vi "WILT Start Stop Timer Set.vi"(4 "Station Number":i32, 6 "Injection Times":T1, 7 "Operation Type":T2=enum."Operate As Stand-Alone EXE", 10 "Inlet Timer":dbl, 11 "Station Test State In":T3) -> (3 "Outlet Timer":dbl)   [LabVIEW 2016]
uses:
  Type Definitions/WILT Station Test State Cluster.ctl
  Type Definitions/WILT Dryer Test State.ctl
  Type Definitions/WILT Water Valve EXE Operation Type.ctl
  Type Definitions/WILT Water Injection Control.ctl
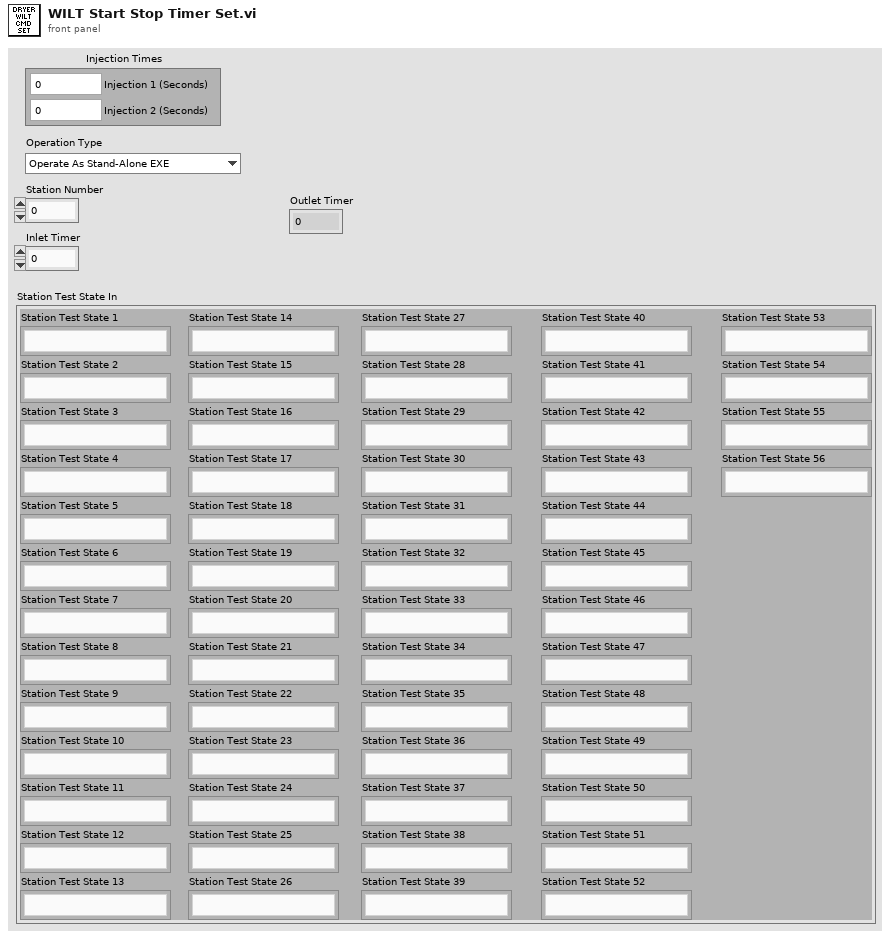
[diagram p1: front panel]
types:
  T1 = typedef "WILT Water Injection Control.ctl" = cluster{"Injection 1 (Seconds)":dbl, "Injection 2 (Seconds)":dbl}
  T2 = typedef "WILT Water Valve EXE Operation Type.ctl" = enum16{"Operate As SubVI", "Operate As Stand-Alone EXE", "Shutdown All Dryers"}
  T3 = typedef "WILT Station Test State Cluster.ctl" = cluster{"Station Test State 1":T4, "Station Test State 2":T4, "Station Test State 3":T4, "Station Test State 4":T4, "Station Test State 5":T4, "Station Test State 6":T4, "Station Test State 7":T4, "Station Test State 8":T4, "Station Test State 9":T4, "Station Test State 10":T4, "Station Test State 11":T4, "Station Test State 12":T4, "Station Test State 13":T4, "Station Test State 14":T4, "Station Test State 15":T4, "Station Test State 16":T4, "Station Test State 17":T4, "Station Test State 18":T4, "Station Test State 19":T4, "Station Test State 20":T4, "Station Test State 21":T4, "Station Test State 22":T4, "Station Test State 23":T4, "Station Test State 24":T4, "Station Test State 25":T4, "Station Test State 26":T4, "Station Test State 27":T4, "Station Test State 28":T4, "Station Test State 29":T4, "Station Test State 30":T4, "Station Test State 31":T4, "Station Test State 32":T4, "Station Test State 33":T4, "Station Test State 34":T4, "Station Test State 35":T4, "Station Test State 36":T4, "Station Test State 37":T4, "Station Test State 38":T4, "Station Test State 39":T4, "Station Test State 40":T4, "Station Test State 41":T4, "Station Test State 42":T4, "Station Test State 43":T4, "Station Test State 44":T4, "Station Test State 45":T4, "Station Test State 46":T4, "Station Test State 47":T4, "Station Test State 48":T4, "Station Test State 49":T4, "Station Test State 50":T4, "Station Test State 51":T4, "Station Test State 52":T4, "Station Test State 53":T4, "Station Test State 54":T4, "Station Test State 55":T4, "Station Test State 56":T4}
  T4 = typedef "WILT Dryer Test State.ctl" = enum16{"No Serial Number", "Waiting for Dryer To Start", "Drying Clothes", "Water Injection 1 (On)", "Water Injection 1 Timer", "Water Injection 1 (Off)", "Pause Dryer", "Sending Start Stop CMD", "Pause Dryer 2", "Sending Start Stop CMD 2", "Drying Clothes 2", "Water Injection 2 (On)", "Water Injection 2 Timer", "Water Injection 2 (Off)", "Drying Clothes 3", "Cooling Down", "Sending Start Stop CMD 3", "Increment Cycle"}
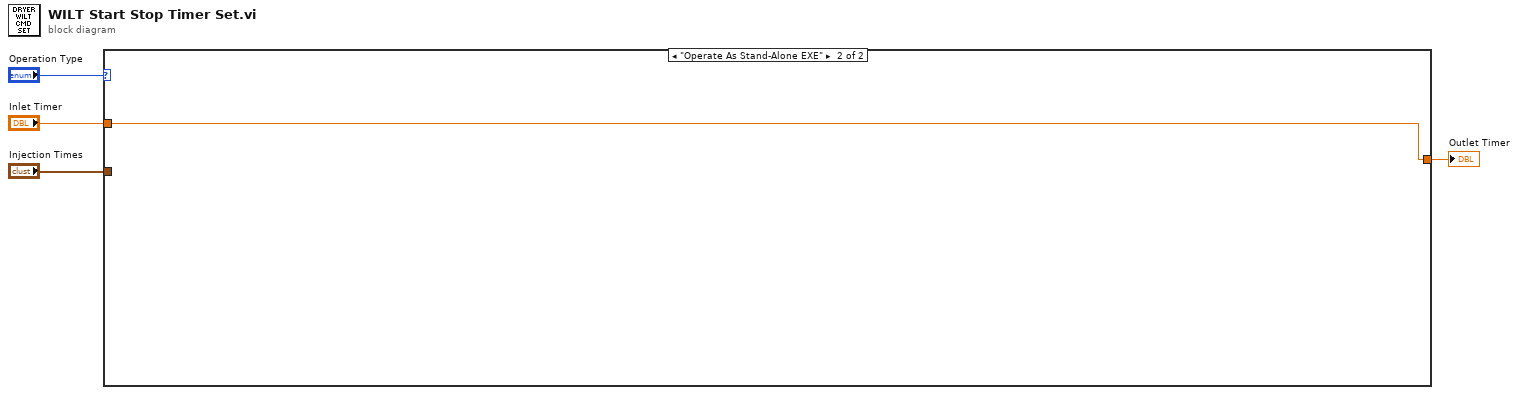
[diagram p0: block diagram]
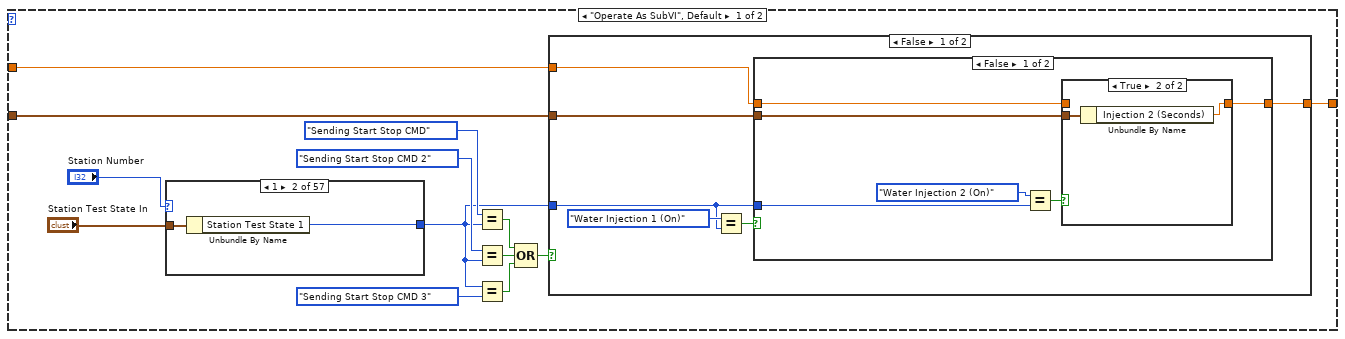
[diagram p2: hidden frame]
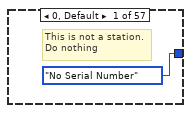
[diagram p3: hidden frame]
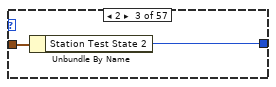
[diagram p4: hidden frame]
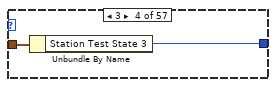
[diagram p5: hidden frame]
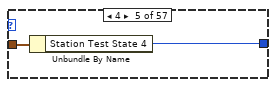
[diagram p6: hidden frame]
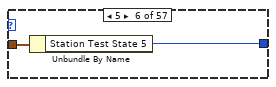
[diagram p7: hidden frame]
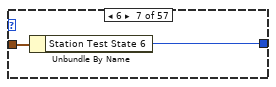
[diagram p8: hidden frame]
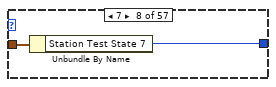
[diagram p9: hidden frame]
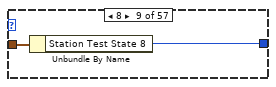
[diagram p10: hidden frame]
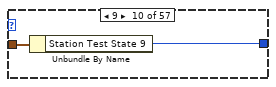
[diagram p11: hidden frame]
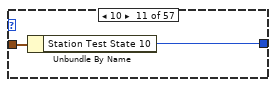
[diagram p12: hidden frame]
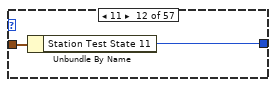
[diagram p13: hidden frame]
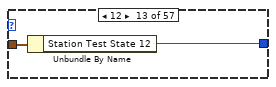
[diagram p14: hidden frame]
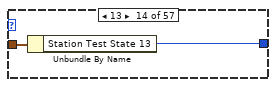
[diagram p15: hidden frame]
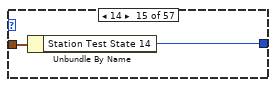
[diagram p16: hidden frame]
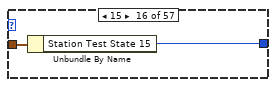
[diagram p17: hidden frame]
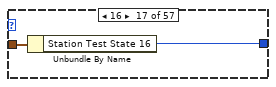
[diagram p18: hidden frame]
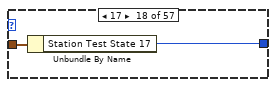
[diagram p19: hidden frame]
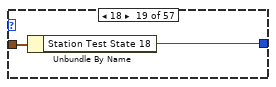
[diagram p20: hidden frame]
diagram:
  n1 = case shown="\"Operate As Stand-Alone EXE\"" "Operation Type" {
    tunnel: "Inlet Timer" -> [w10 w149]
    tunnel: [w9 w149] -> w3
    tunnel: "Injection Times" -> [w5 _]
    frame "Operate As SubVI", Default {
      n2 = case shown="1" "Station Number" {
        tunnel: "Station Test State In" -> [_ w20 w22 w24 w26 w28 w30 w32 w34 w36 w38 w40 w42 w44 w46 w48 w50 w52 w54 w56 w58 w60 w62 w64 w66 w68 w70 w72 w74 w76 w78 w80 w82 w84 w86 w88 w90 w92 w94 w96 w98 w100 w102 w104 w106 w108 w110 w112 w114 w116 w118 w120 w122 w124 w126 w128 w130]
        tunnel: [WILT_Dryer_Test_State."No Serial Number" ("Station Test State 56") w19 w21 w23 w25 w27 w29 w31 w33 w35 w37 w39 w41 w43 w45 w47 w49 w51 w53 w55 w57 w59 w61 w63 w65 w67 w69 w71 w73 w75 w77 w79 w81 w83 w85 w87 w89 w91 w93 w95 w97 w99 w101 w103 w105 w107 w109 w111 w113 w115 w117 w119 w121 w123 w125 w127 w129] -> w6
        frame 0, Default {
          # "This is not a station.\nDo nothing"
        }
        frame 1 {
          n3 = Unbundle By Name(w20) -> ("Station Test State 1"=w19:T4)
        }
        frame 2 {
          n4 = Unbundle By Name(w22) -> ("Station Test State 2"=w21:T4)
        }
        frame 3 {
          n5 = Unbundle By Name(w24) -> ("Station Test State 3"=w23:T4)
        }
        frame 4 {
          n6 = Unbundle By Name(w26) -> ("Station Test State 4"=w25:T4)
        }
        frame 5 {
          n7 = Unbundle By Name(w28) -> ("Station Test State 5"=w27:T4)
        }
        frame 6 {
          n8 = Unbundle By Name(w30) -> ("Station Test State 6"=w29:T4)
        }
        frame 7 {
          n9 = Unbundle By Name(w32) -> ("Station Test State 7"=w31:T4)
        }
        frame 8 {
          n10 = Unbundle By Name(w34) -> ("Station Test State 8"=w33:T4)
        }
        frame 9 {
          n11 = Unbundle By Name(w36) -> ("Station Test State 9"=w35:T4)
        }
        frame 10 {
          n12 = Unbundle By Name(w38) -> ("Station Test State 10"=w37:T4)
        }
        frame 11 {
          n13 = Unbundle By Name(w40) -> ("Station Test State 11"=w39:T4)
        }
        frame 12 {
          n14 = Unbundle By Name(w42) -> ("Station Test State 12"=w41:T4)
        }
        frame 13 {
          n15 = Unbundle By Name(w44) -> ("Station Test State 13"=w43:T4)
        }
        frame 14 {
          n16 = Unbundle By Name(w46) -> ("Station Test State 14"=w45:T4)
        }
        frame 15 {
          n17 = Unbundle By Name(w48) -> ("Station Test State 15"=w47:T4)
        }
        frame 16 {
          n18 = Unbundle By Name(w50) -> ("Station Test State 16"=w49:T4)
        }
        frame 17 {
          n19 = Unbundle By Name(w52) -> ("Station Test State 17"=w51:T4)
        }
        frame 18 {
          n20 = Unbundle By Name(w54) -> ("Station Test State 18"=w53:T4)
        }
        frame 19 {
          n21 = Unbundle By Name(w56) -> ("Station Test State 19"=w55:T4)
        }
        frame 20 {
          n22 = Unbundle By Name(w58) -> ("Station Test State 20"=w57:T4)
        }
        frame 21 {
          n23 = Unbundle By Name(w60) -> ("Station Test State 21"=w59:T4)
        }
        frame 22 {
          n24 = Unbundle By Name(w62) -> ("Station Test State 22"=w61:T4)
        }
        frame 23 {
          n25 = Unbundle By Name(w64) -> ("Station Test State 23"=w63:T4)
        }
        frame 24 {
          n26 = Unbundle By Name(w66) -> ("Station Test State 24"=w65:T4)
        }
        frame 25 {
          n27 = Unbundle By Name(w68) -> ("Station Test State 25"=w67:T4)
        }
        frame 26 {
          n28 = Unbundle By Name(w70) -> ("Station Test State 26"=w69:T4)
        }
        frame 27 {
          n29 = Unbundle By Name(w72) -> ("Station Test State 27"=w71:T4)
        }
        frame 28 {
          n30 = Unbundle By Name(w74) -> ("Station Test State 28"=w73:T4)
        }
        frame 29 {
          n31 = Unbundle By Name(w76) -> ("Station Test State 29"=w75:T4)
        }
        frame 30 {
          n32 = Unbundle By Name(w78) -> ("Station Test State 30"=w77:T4)
        }
        frame 31 {
          n33 = Unbundle By Name(w80) -> ("Station Test State 31"=w79:T4)
        }
        frame 32 {
          n34 = Unbundle By Name(w82) -> ("Station Test State 32"=w81:T4)
        }
        frame 33 {
          n35 = Unbundle By Name(w84) -> ("Station Test State 33"=w83:T4)
        }
        frame 34 {
          n36 = Unbundle By Name(w86) -> ("Station Test State 34"=w85:T4)
        }
        frame 35 {
          n37 = Unbundle By Name(w88) -> ("Station Test State 35"=w87:T4)
        }
        frame 36 {
          n38 = Unbundle By Name(w90) -> ("Station Test State 36"=w89:T4)
        }
        frame 37 {
          n39 = Unbundle By Name(w92) -> ("Station Test State 37"=w91:T4)
        }
        frame 38 {
          n40 = Unbundle By Name(w94) -> ("Station Test State 38"=w93:T4)
        }
        frame 39 {
          n41 = Unbundle By Name(w96) -> ("Station Test State 39"=w95:T4)
        }
        frame 40 {
          n42 = Unbundle By Name(w98) -> ("Station Test State 40"=w97:T4)
        }
        frame 41 {
          n43 = Unbundle By Name(w100) -> ("Station Test State 41"=w99:T4)
        }
        frame 42 {
          n44 = Unbundle By Name(w102) -> ("Station Test State 42"=w101:T4)
        }
        frame 43 {
          n45 = Unbundle By Name(w104) -> ("Station Test State 43"=w103:T4)
        }
        frame 44 {
          n46 = Unbundle By Name(w106) -> ("Station Test State 44"=w105:T4)
        }
        frame 45 {
          n47 = Unbundle By Name(w108) -> ("Station Test State 45"=w107:T4)
        }
        frame 46 {
          n48 = Unbundle By Name(w110) -> ("Station Test State 46"=w109:T4)
        }
        frame 47 {
          n49 = Unbundle By Name(w112) -> ("Station Test State 47"=w111:T4)
        }
        frame 48 {
          n50 = Unbundle By Name(w114) -> ("Station Test State 48"=w113:T4)
        }
        frame 49 {
          n51 = Unbundle By Name(w116) -> ("Station Test State 49"=w115:T4)
        }
        frame 50 {
          n52 = Unbundle By Name(w118) -> ("Station Test State 50"=w117:T4)
        }
        frame 51 {
          n53 = Unbundle By Name(w120) -> ("Station Test State 51"=w119:T4)
        }
        frame 52 {
          n54 = Unbundle By Name(w122) -> ("Station Test State 52"=w121:T4)
        }
        frame 53 {
          n55 = Unbundle By Name(w124) -> ("Station Test State 53"=w123:T4)
        }
        frame 54 {
          n56 = Unbundle By Name(w126) -> ("Station Test State 54"=w125:T4)
        }
        frame 55 {
          n57 = Unbundle By Name(w128) -> ("Station Test State 55"=w127:T4)
        }
        frame 56 {
          n58 = Unbundle By Name(w130) -> ("Station Test State 56"=w129:T4)
        }
      }
      n59 = Equal?(x=WILT_Dryer_Test_State."Sending Start Stop CMD", y=w6) -> (x = y?=w14:bool)
      n60 = Equal?(x=WILT_Dryer_Test_State."Sending Start Stop CMD 2", y=w6) -> (x = y?=w13:bool)
      n61 = Equal?(x=w6, y=WILT_Dryer_Test_State."Sending Start Stop CMD 3" ("x")) -> (x = y?=w12:bool)
      n62 = Compound Arithmetic op=OR(w14, w13, w12) -> (w11:bool)
      n63 = case shown="False" w11 {
        tunnel: [w132 500.0] -> w9
        tunnel: w10 -> [w133 _]
        tunnel: w6 -> [w131 _]
        tunnel: w5 -> [w134 _]
        frame False {
          n64 = Equal?(x=WILT_Dryer_Test_State."Water Injection 1 (On)", y=w131) -> (x = y?=w135:bool)
          n65 = case shown="False" w135 {
            tunnel: w134 -> [w139 w147]
            tunnel: w133 -> [w137 _]
            tunnel: [w138 w146] -> w132
            tunnel: w131 -> [w141 _]
            frame False {
              n66 = Equal?(x=WILT_Dryer_Test_State."Water Injection 2 (On)", y=w141) -> (x = y?=w140:bool)
              n67 = case shown="True" w140 {
                tunnel: w139 -> [_ w145]
                tunnel: [w143 w144] -> w138
                tunnel: w137 -> [w143 _]
                frame False {
                }
                frame True {
                  n68 = Unbundle By Name(w145) -> ("Injection 2 (Seconds)"=w144:dbl)
                }
              }
            }
            frame True {
              n69 = Unbundle By Name(w147) -> ("Injection 1 (Seconds)"=w146:dbl)
            }
          }
        }
        frame True {
          # "Cycle Time for Start\nStop buttons"
        }
      }
    }
    frame "Operate As Stand-Alone EXE" {
    }
  }
  "Outlet Timer" <- w3
